vi "Write Draw Animation.vi"(8 "error in (no error)":errorcluster, 9 "Draw Animation?":bool, 11 "3D Comet.lvclass in":refnum<class "3D Comet.lvclass">) -> (0 "error out":errorcluster, 3 "3D Comet.lvclass out":refnum<class "3D Comet.lvclass">)   [LabVIEW 2020, in "3D Comet.lvclass"]
uses:
  <vilib>/Math Plots/3D Math Plots/3D Comet/3D Comet/3D Comet.lvclass
  <vilib>/Math Plots/3D Math Plots/3D Comet/3D Comet/3D Comet.lvclass/3D Comet.ctl
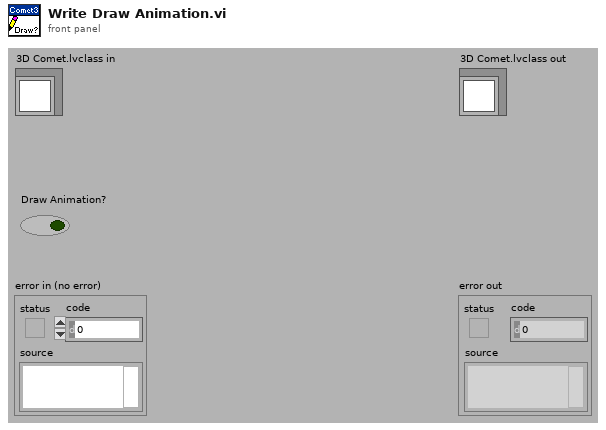
[diagram p1: front panel]
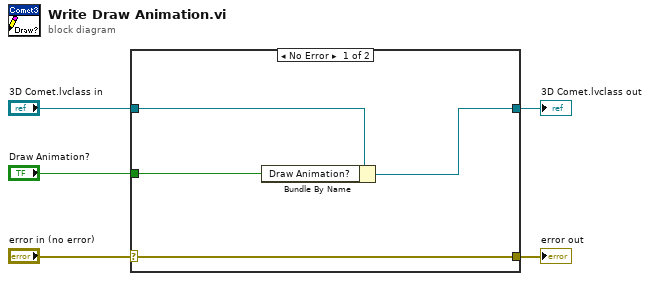
[diagram p0: block diagram]
diagram:
  n1 = case shown="No Error" "error in (no error)" {
    selector: "error in (no error)" -> [w9 w10]
    tunnel: [w9 w10] -> w4
    tunnel: [w7 w11] -> w2
    tunnel: "3D Comet.lvclass in" -> [w8 w11]
    tunnel: "Draw Animation?" -> [w6 _]
    frame No Error {
      n2 = Bundle By Name(cluster=w8, "Draw Animation?"=w6) -> (w7:refnum<class "3D Comet.lvclass">)
    }
    frame Error {
    }
  }
  "error out" <- w4
  "3D Comet.lvclass out" <- w2
